vi "(TestVI)Get BD Info.vi"() -> ()   [LabVIEW 2020]
uses:
  SubVIs/Serial/Controls/(Ctrl)Serial_FGV Function.ctl
panel:
  out "BD Version":T1 {"BD FW Version" format="%08x"}
  in  "VISA resource name":refnum<visa-resource-name>
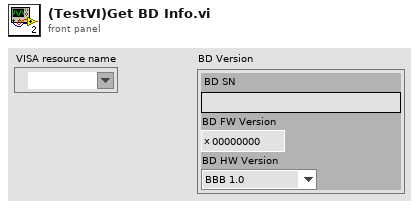
[diagram p1: front panel]
types:
  T1 = cluster{"BD SN":string, "BD FW Version":u32, "BD HW Version":enum8{"BBB 1.0", "BBB 1.1", "WBB 1.0", "reserved", "RedNoah3"}}
  T2 = typedef "(Ctrl)Serial_FGV Function.ctl" = enum16{"Initialize", "Read", "Read All", "Write", "Flush Buffer", "Get Ref.", "Close"}
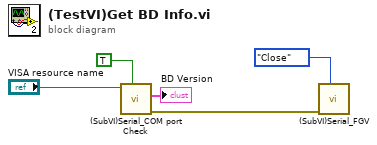
[diagram p0: block diagram]
diagram:
  n1 = call "(SubVI)Serial_COM port Check.vi"("Auto Detect?"=TRUE, "VISA resource name"="VISA resource name") -> ("error out"=w2:errorcluster, "BD Version"=→"BD Version":T1)  [unwired: 3 in, 5 out]
  n2 = call "(SubVI)Serial_FGV.vi"("Function"=(Ctrl)Serial_FGV_Function."Close", "error in (no error)"=w2) -> ()  [unwired: 7 in, 3 out]
